vi "Open CSM BD.vi"(7 "Current Module(\"\" to generate a ID)":string, 8 "error in (no error)":errorcluster, 11 "CSM":string) -> (0 "error out":errorcluster)   [LabVIEW 2017, in "csm-tool-support.lvlib"]
doc: "-- <b>Controls</b> --\n- <b>Current Module(\"\" to generate a ID)</b>:\n- <b>CSM</b>:"
uses:
  csm-tool-support.lvlib
  _csmHelper/API with lvcsm Support/CSM-Helper API with lvcsm Support.lvlib
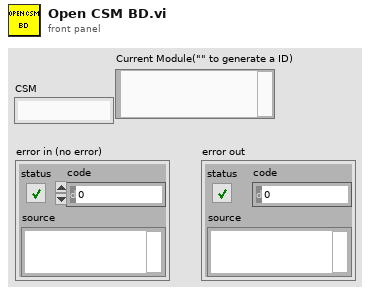
[diagram p1: front panel]
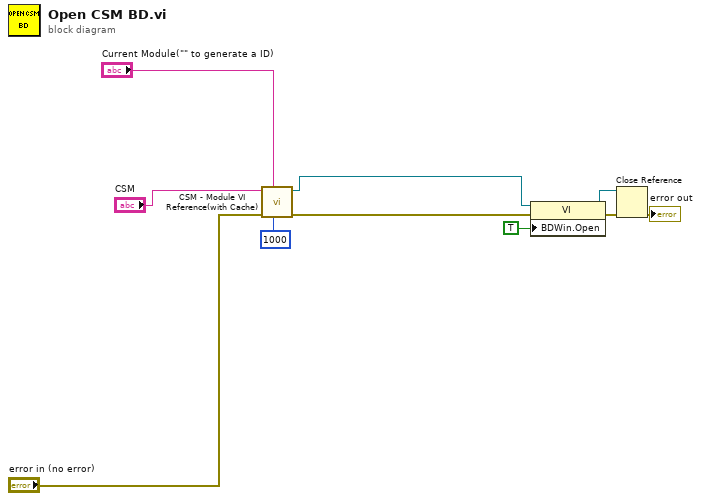
[diagram p0: block diagram]
diagram:
  n1 = call "CSM - Module VI Reference(with Cache).vi"("Response Timeout(-2 using Global Settings)"=1000 ("Response Timeout(5000ms)"), "Current Module(\"\" to generate a ID)"="Current Module(\"\" to generate a ID)", "error in (no error)"="error in (no error)", "CSM Name"="CSM") -> ("error out"=w9:errorcluster, "CSM Module VIRef"=w1:refnum<vi>)  [unwired: 6 in]
  n2 = property class="VI"(reference=w1, error in=w9, "BDWin.Open"=TRUE ("Block Diagram Window:Open")) -> (reference out=w5:refnum<vi>, error out=w7:errorcluster)
  n3 = Close Reference(reference=w5, error in (no error)=w7) -> (error out=→"error out":errorcluster)
